vi "Initialize.vi"(7 "rows (auto from ref)":i32=-1, 8 "error in (no error)":errorcluster, 9 "# columns":i32=1 caption="Number of columns", 10 "Add Timestamp? (T)":bool=TRUE, 11 "Table":refnum<vi>) -> (0 "error out":errorcluster, 3 "Cyclic Table":refnum<class "Cyclic Table.lvclass">)   [LabVIEW 2024, in "Cyclic Table.lvclass"]
doc: "Initialize the Cyclic Table. This is a circular buffer for arrays of strings. The number of columns is input (arrays entered with more column will be truncated). The number of rows is matched to the number of visible rows in the entered Table control."
uses:
  Cyclic Table.lvclass
  Cyclic Table.lvclass/Cyclic Table.ctl
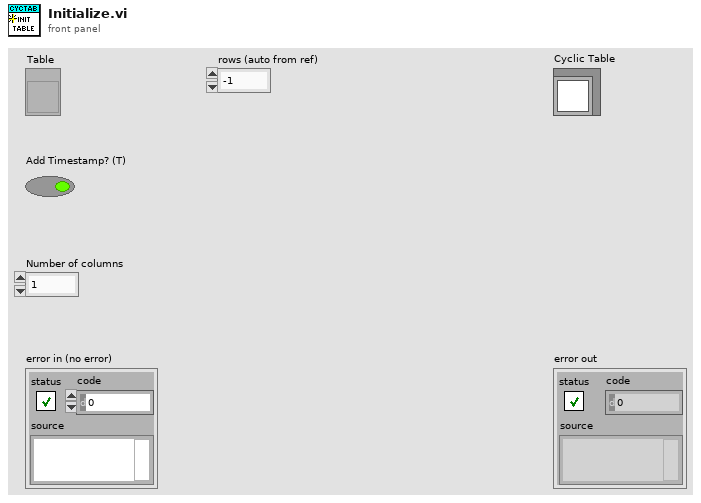
[diagram p1: front panel]
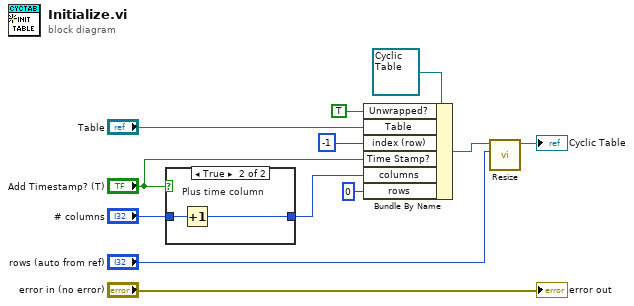
[diagram p0: block diagram]
diagram:
  n1 = case shown="True" "Add Timestamp? (T)" {
    tunnel: "# columns" -> [w13 w15]
    tunnel: [w13 w14] -> w9
    frame False {
    }
    frame True {
      n2 = Increment "Plus time column"(x=w15) -> (x+1=w14:i32)
    }
  }
  n3 = Bundle By Name(cluster=refnum<class "Cyclic Table.lvclass"> refnum ("Cyclic Table in"), "Unwrapped?"=TRUE, "Table"="Table", "index (row)"=-1, "Time Stamp?"="Add Timestamp? (T)", "columns"=w9, "rows"=0) -> (w8:refnum<class "Cyclic Table.lvclass">)
  n4 = call "Resize.vi"("Number of Rows (auto from ref)"="rows (auto from ref)", "Cyclic Table in"=w8) -> ("Cyclic Table out"=→"Cyclic Table":refnum<class "Cyclic Table.lvclass">)  [unwired: 9 in]
  "error out" <- "error in (no error)"
